vi "Error Query.vi"(8 "error in (no error)":errorcluster, 9 "clear error register (T:yes)":bool=TRUE, 11 "VISA resource name":refnum<visa-resource-name>) -> (0 "error out":errorcluster, 1 "error message":string, 2 "error":bool, 3 "VISA resource name out":refnum<visa-resource-name>)   [LabVIEW 2017, in "Fluke 8840.lvlib"]
doc: "This VI reads an error from the instrument."
uses:
  Fluke 8840.lvlib
panel:
  # "yes\nno"
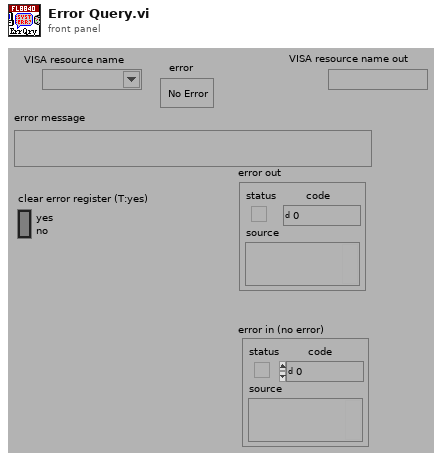
[diagram p1: front panel]
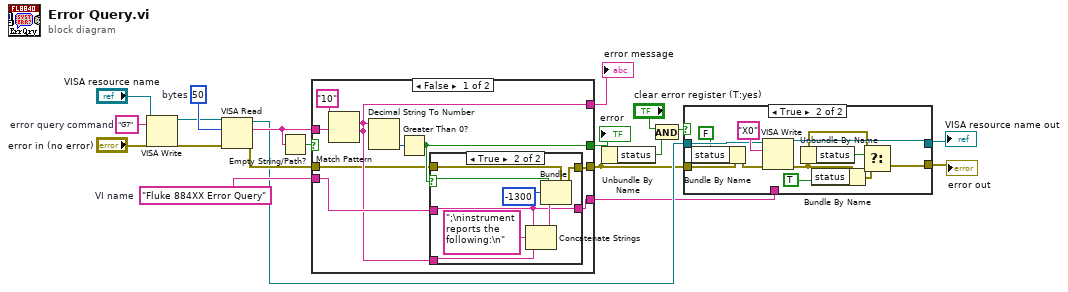
[diagram p0: block diagram]
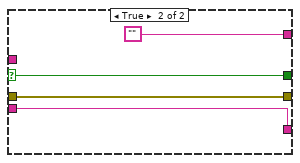
[diagram p4: hidden frame]
diagram:
  w16 = u32 50  # bytes
  w19 = "G7"  # error query command
  w12 = "Fluke 884XX Error Query"  # VI name
  n1 = VISA Write(VISA resource name="VISA resource name", write buffer=w19, error in (no error)="error in (no error)") -> (VISA resource name out=w15:refnum<visa-resource-name>, error out=w18:errorcluster)  [unwired: 1 out]
  n2 = VISA Read(VISA resource name=w15, byte count=w16, error in (no error)=w18) -> (VISA resource name out=w8:refnum<visa-resource-name>, read buffer=w10:string, error out=w11:errorcluster)  [unwired: 1 out]
  n3 = Empty String/Path?(string/path=w10) -> (empty?=w9:bool)
  n4 = case shown="False" w9 {
    selector: w9 -> [_ w42]
    tunnel: w10 -> [w28 _]
    tunnel: w11 -> [w22 w43]
    tunnel: [w21 w43] -> w1
    tunnel: [w26 w42] -> w14
    tunnel: [w23 ""] -> w13
    tunnel: w12 -> [w25 w40]
    tunnel: [w24 w40] -> w5
    frame False {
      n5 = Match Pattern(string=w28, regular expression="10") -> (after substring=w23:string)  [unwired: 4 out]
      n6 = Decimal String To Number(string=w23) -> (number=w29:i32)  [unwired: 3 out]
      n7 = Greater Than 0?(x=w29) -> (x > 0?=w26:bool)
      n8 = case shown="True" w26 {
        selector: w26 -> [_ w34]
        tunnel: w25 -> [w30 w36]
        tunnel: [w30 w36] -> w24
        tunnel: w23 -> [_ w35]
        tunnel: w22 -> [w31 w33]
        tunnel: [w31 w32] -> w21
        frame False {
        }
        frame True {
          n9 = Concatenate Strings(w36, ";\ninstrument reports the following:\n", w35) -> (w39:string)
          n10 = Bundle(cluster=w33, "status"=w34, "code"=-1300, "source"=w39) -> (w32:errorcluster)
        }
      }
    }
    frame True {
    }
  }
  "error message" <- w13
  "error" <- w14
  n11 = Unbundle By Name(w1) -> ("status"=w4:bool)
  n12 = And(x="clear error register (T:yes)", y=w4) -> (x .and. y?=w2:bool)
  n13 = case shown="True" w2 {
    tunnel: w1 -> [w44 w47]
    tunnel: w8 -> [w45 w55]
    tunnel: [w45 w54] -> w7
    tunnel: [w44 w48] -> w6
    tunnel: w5 -> [_ _]
    frame False {
    }
    frame True {
      n14 = Bundle By Name(cluster=w47, "status"=FALSE) -> (w46:errorcluster)
      n15 = VISA Write(VISA resource name=w55, write buffer="X0", error in (no error)=w46) -> (VISA resource name out=w54:refnum<visa-resource-name>, error out=w51:errorcluster)  [unwired: 1 out]
      n16 = Unbundle By Name(w51) -> ("status"=w52:bool)
      n17 = Bundle By Name(cluster=w51, "status"=TRUE) -> (w50:errorcluster)
      n18 = Select(t=w51, s=w52, f=w50) -> (s? t:f=w48:errorcluster)
    }
  }
  "error out" <- w6
  "VISA resource name out" <- w7
